vi "subStage_GotoAccordingtoTable.vi"(7 "Record Table":string[][](table), 8 "error in (no error)":errorcluster, 10 "ILSID":i32=1, 11 "Number":dbl) -> (0 "error out":errorcluster)   [LabVIEW 2015]
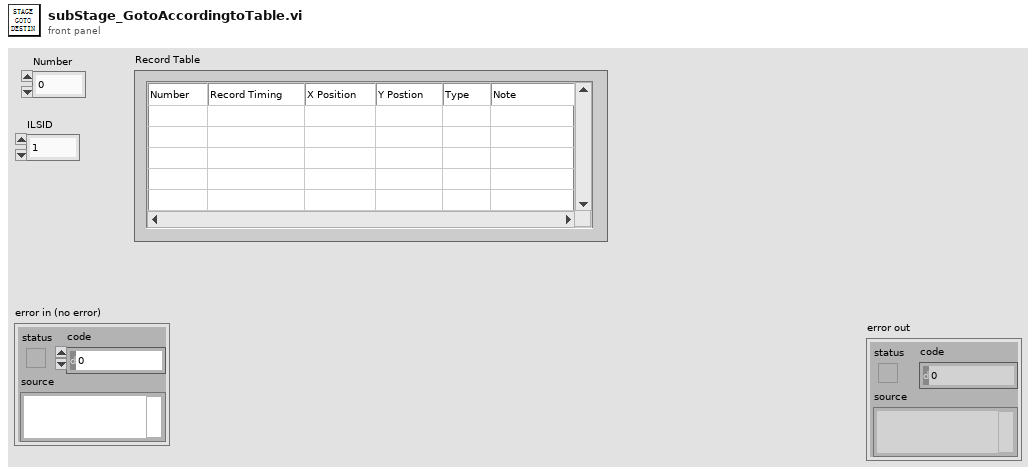
[diagram p1: front panel]
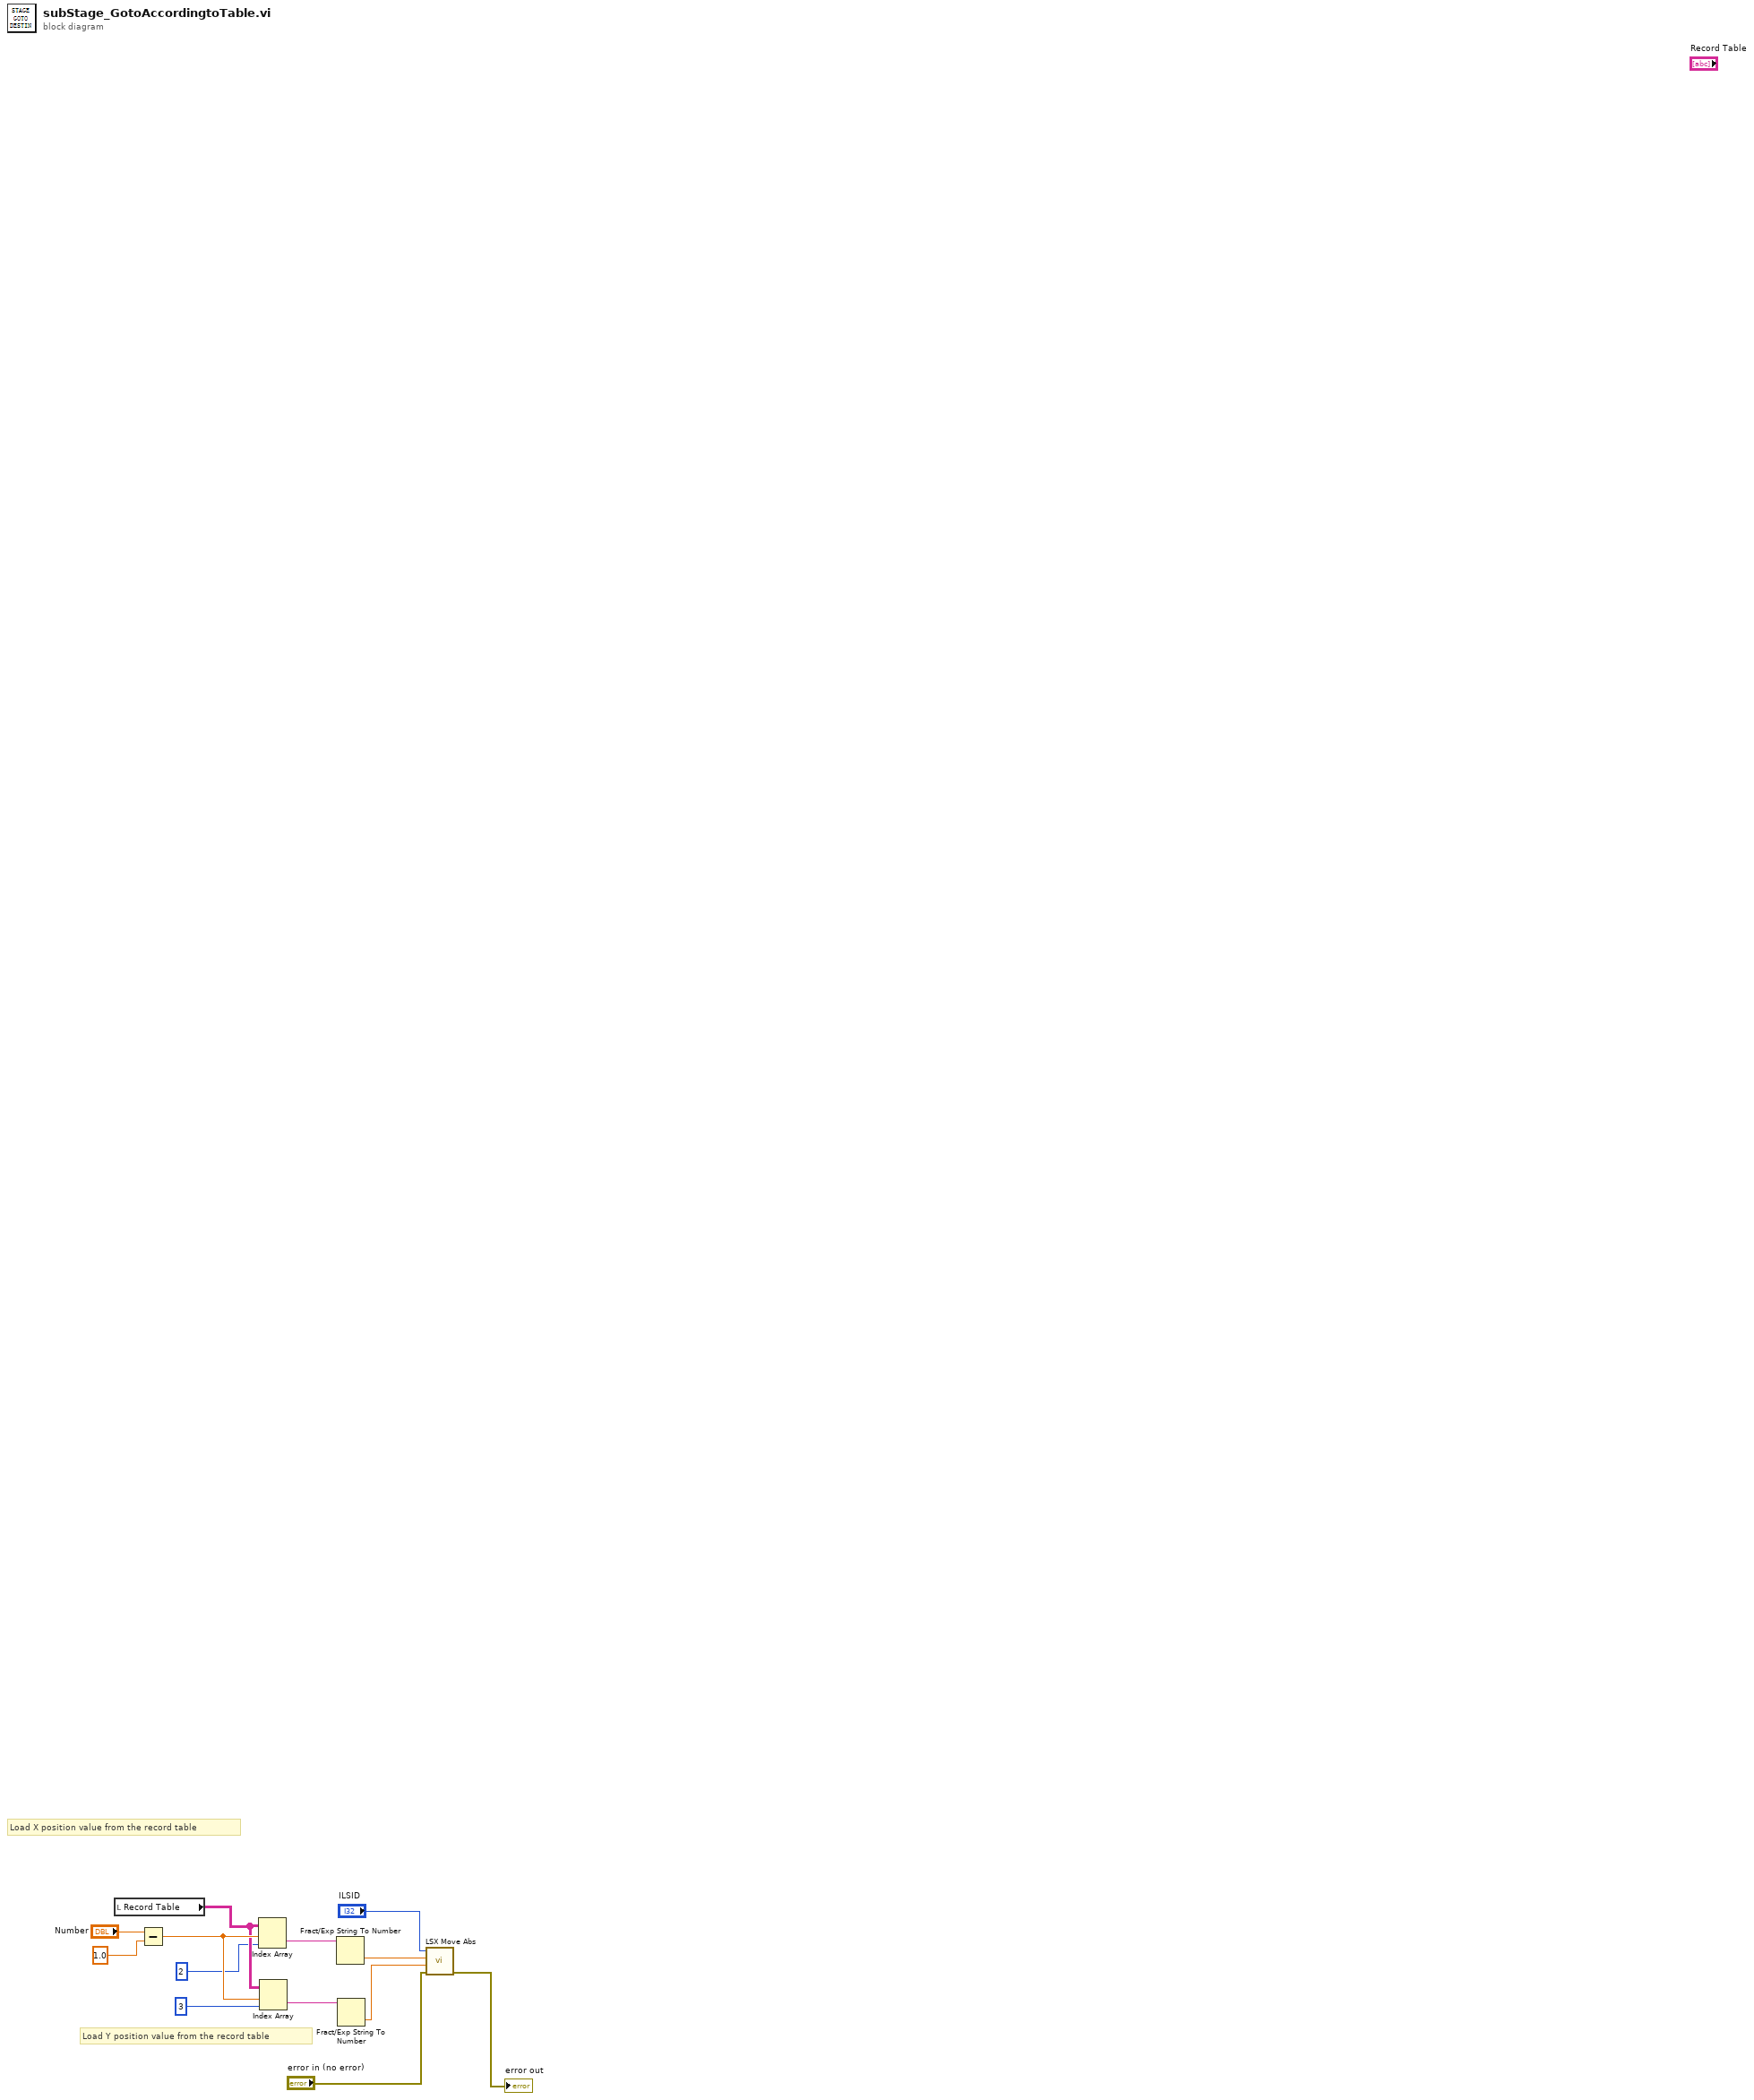
[diagram p0: block diagram]
diagram:
  # "Load Y position value from the record table"
  # "Load X position value from the record table"
  n1 = local read "Record Table"() -> (w5:string[][])
  n2 = Subtract(x="Number", y=1.0) -> (x-y=w13:dbl)
  n3 = Index Array(array=w5, index (row)=w13, index (col)=2 ("disabled index (col)")) -> (element=w7:string)
  n4 = Index Array(array=w5, index (row)=w13, index (col)=3 ("disabled index (col)")) -> (element=w9:string)
  n5 = Fract/Exp String To Number(string=w7) -> (number=w8:dbl)  [unwired: 3 in, 1 out]
  n6 = Fract/Exp String To Number(string=w9) -> (number=w10:dbl)  [unwired: 3 in, 1 out]
  n7 = call <userlib>:"LSX Move Abs.vi"("error in (no error)"="error in (no error)", "dY"=w10, "dX"=w8, "lLSID"="ILSID") -> ("error out"=→"error out":errorcluster)  [unwired: 6 in, 1 out]
